vi "Trig OP Setup-Gen keys array.vi"(11 "Trigger index (FOR loop index)":i32) -> (3 "Keys array for each trigger":string[](array[string]))   [LabVIEW 2020]
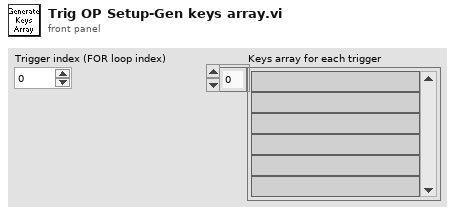
[diagram p1: front panel]
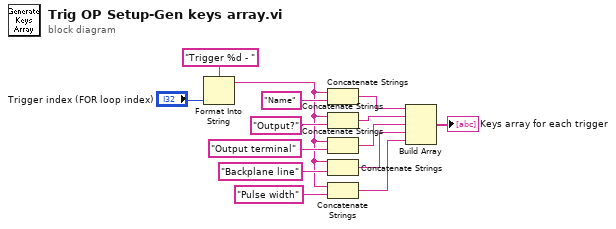
[diagram p0: block diagram]
diagram:
  n1 = Format Into String(format string="Trigger %d - ", "Trigger index (FOR loop index)") -> (resulting string=w2:string)  [unwired: 2 in, 1 out]
  n2 = Concatenate Strings(w2, "Name" ("string")) -> (w9:string)
  n3 = Concatenate Strings(w2, "Output?" ("string")) -> (w10:string)
  n4 = Concatenate Strings(w2, "Output terminal" ("string")) -> (w11:string)
  n5 = Concatenate Strings(w2, "Backplane line" ("string")) -> (w12:string)
  n6 = Concatenate Strings(w2, "Pulse width" ("string")) -> (w1:string)
  n7 = Build Array(w9, w10, w11, w12, w1) -> (→"Keys array for each trigger":string[])
